vi "FRC_Scout.vi"() -> ()   [LabVIEW 2013]
doc: "The Grab (Express) VI acquires images continuously and displays the images in an image control using the Vision Acquisition Express VI. A grab is appropriate for high-speed applications in which you need to process only one image at a time."
uses:
  <vilib>/vision/Instrument.llb/QR Code Search Options.ctl
  <vilib>/vision/Instrument.llb/Demodulation Mode.ctl
  <vilib>/vision/Instrument.llb/Cell Sample Size.ctl
  <vilib>/vision/Instrument.llb/Cell Filter Mode.ctl
  <vilib>/vision/Instrument.llb/QR Code Description Options.ctl
  <vilib>/vision/Instrument.llb/Data Matrix Polarity.ctl
  <vilib>/vision/Instrument.llb/QR Code Model Type.ctl
  Instance           1 22Saved   Grab (Express) .vi
  <vilib>/LVH/i3 JSON/JSON Generation/Create Value Files/Create Value - Object.vi
  <vilib>/LVH/i3 JSON/JSON Generation/Add Object Parameter Files/Add Object Parameter - Object.vi
  <vilib>/LVH/i3 JSON/JSON Parsing/Get Object Parameter Files/Get Object Parameter - Object.vi
  <vilib>/vision/NI_Vision_Development_Module.lvlib
  <vilib>/LVH/i3 JSON/i3-json.lvlib
panel:
  out "Header":string
  out "Scores":T1
  out "Auto":T2
  out "Team":T3
  in  "QR Tab Control":T4(tab)
  in  "Auto Comments":string="How did autonomous work?"
  in  "T Stack":bool
  in  "B Mov":bool
  in  "T Mov":bool
  in  "Can PU Rec Bin":bool
  in  "Can PU Tote":bool
  in  "Can PU Noodles":bool
  in  "Drive Train":u16(ring) items=["Standard Wheels", "Omni Wheels", "Mecanum Wheels", "Swerve Drive"]
  in  "Comments":string="What else do we need to know?"
  in  "Max Tote":u8
  in  "Match":string="0"
  in  "Team #":u16
  in  "0":u8
  in  "1":u8
  in  "4":u8
  in  "2":u8
  in  "6A":u8
  in  "6B":u8
  in  "Inc0":bool
  in  "Inc1":bool
  in  "Inc2":bool
  in  "Inc4":bool
  in  "Inc6A":bool
  in  "Inc6B":bool
  in  "6C":u8
  in  "8":u8
  in  "10":u8
  in  "12A":u8
  in  "12B":u8
  in  "12C":u8
  in  "18A":u8
  in  "18B":u8
  in  "20":u8
  in  "24A":u8
  in  "24B":u8
  in  "30A":u8
  in  "30B":u8
  in  "36A":u8
  in  "36B":u8
  in  "40":u8
  in  "42":u8
  in  "Inc6C":bool
  in  "Inc8":bool
  in  "Inc10":bool
  in  "Inc12A":bool
  in  "Inc12B":bool
  in  "Inc12C":bool
  in  "Inc18B":bool
  in  "Inc18A":bool
  in  "Inc20":bool
  in  "Inc24A":bool
  in  "Inc24B":bool
  in  "Inc30A":bool
  in  "Inc30B":bool
  in  "Inc36A":bool
  in  "Inc36B":bool
  in  "Inc40":bool
  in  "Inc42":bool
  in  "Mov":bool
  out "Text Size":i32
  in  "Save  JSON":bool
  in  "Save Image":bool
  out "QR Code":picture
  out "output array":i8[][](array[numeric])
  in  "Export":enum16{"Off", "PNG", "EPS", "JPG"}(ring)=enum."JPG"
  in  "String":string
  in  "Stop Button":bool
  in  "Read New":bool
  out "Frame Rate":dbl
  out "Image":T5(plugin-control)
  out "Buffer Number":u32
  out "Message":string
  out "Read Time (ms)":dbl format="%.2f"
  out "QR Code \nfound":bool
  out "Valid \nRecord":bool
  in  "Save":bool
  out "Team":u16
  out "Match":string
  in  "Assemble and Save":bool
  out "File Number":i32
  in  "Stop":bool
  # "Match"
  # "No QR Code can be produced if \n                  is larger than 2740"
  # "Can pickup:"
  # "Robot Features"
  # "Scoring"
  # "Autonomous"
  # "Moved"
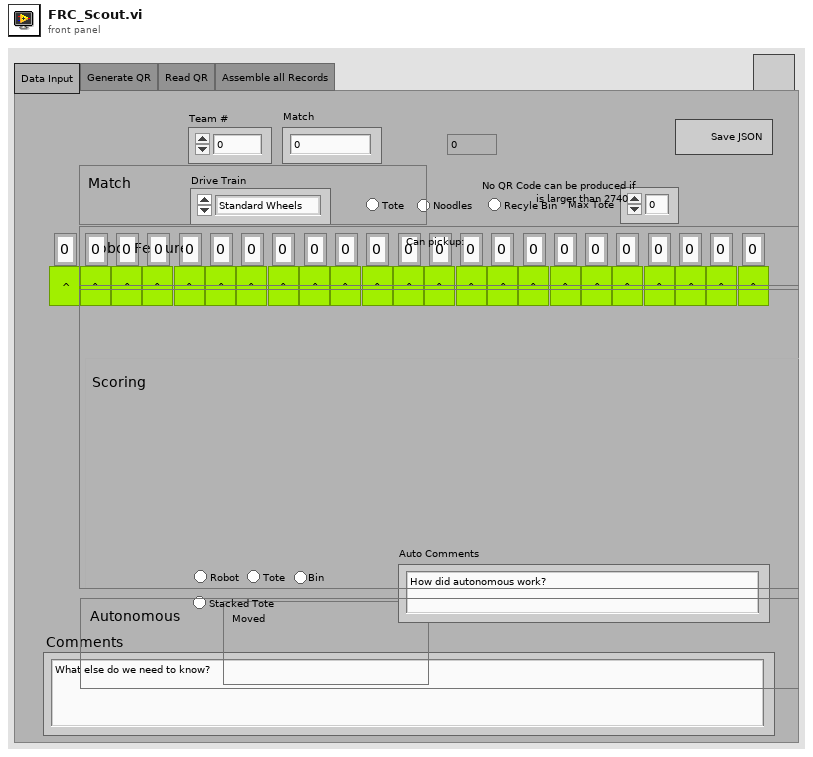
[diagram p1: front panel]
types:
  T1 = cluster{"0":u8, "1":u8, "2":u8, "4":u8, "6A":u8, "6B":u8, "6C":u8, "8":u8, "10":u8, "12A":u8, "12B":u8, "12C":u8, "18A":u8, "18B":u8, "20":u8, "24A":u8, "24B":u8, "30A":u8, "30B":u8, "36A":u8, "36B":u8, "40":u8, "42":u8}
  T2 = cluster{"Robot":bool, "Tote":bool, "Bin":bool, "Tote Stack":bool, "Auto Com":string}
  T3 = cluster{"Unique":string, "Team #":u16, "Match":string, "Max Tote":u8, "Drive":u16, "Noodles":bool, "Tote":bool, "Recylce Bin":bool, "Com":string}
  T4 = enum32{"Data Input", "Generate QR", "Read QR", "Assemble all Records"}
  T5 = typedef "IMAQ Image.ctl" = refnum<image>
  T6 = enum16{"Auto", "1", "2", "3", "4", "5", "6", "7", "8", "9", "10", "11", "12", "13", "14", "15", "16", "17", "18", "19", "20", "21", "22", "23", "24", "25", "26", "27", "28", "29", "30", "31", "32", "33", "34", "35", "36", "37", "38", "39", "40"}
  T7 = enum16{"Numeric", "Alphanumeric", "Binary", "Japanese"}
  T8 = typedef "Image Type" = u32
  T9 = typedef "QR Code Description Options.ctl" = cluster{"Matrix Size (cells)":i32, "Barcode Polarity":T10, "Mirror Mode":i32, "QR Model":T11}
  T10 = typedef "Data Matrix Polarity.ctl" = i32
  T11 = typedef "QR Code Model Type.ctl" = i32
  T12 = typedef "QR Code Search Options.ctl" = cluster{"Rotation Mode":enum32{"Unlimited", "0 Degrees", "90 Degrees", "180 Degrees", "270 Degrees"}, "Skip Location?":bool, "Edge Threshold":u32, "Demodulation Mode":T13, "Cell Sample Size":T14, "Cell Filter Mode":T15, "Skew Degrees Allowed":u32}
  T13 = typedef "Demodulation Mode.ctl" = i32
  T14 = typedef "Cell Sample Size.ctl" = i32
  T15 = typedef "Cell Filter Mode.ctl" = i32
  T16 = typedef "QR Code Report.ctl" = cluster{"Found?":bool, "Data":string, "Bounding Box":cluster{"x":sgl, "y":sgl}[], "Errors Corrected":u32, "Dimensions (Rows/Cols)":u32, "Version":u32, "QR Model":T11, "Stream Mode":T17, "Barcode Polarity":T10, "Mirrored?":bool, "Append Stream Position":u32, "Size of Append Stream":u32, "First EAN-128 ID":i32, "First Alternate Language ID":i32, "Append Stream ID":u32, "Minimum Edge Strength":u32, "Demodulation Mode":T13, "Cell Sample Size":T14, "Cell Filter Mode":T15}
  T17 = typedef "QR Code Stream Mode Type.ctl" = i32
  T18 = cluster{"Unique":string, "Team #":u16, "Match":string, "Max Tote":u8, "Drive Train":u16, "Can PU Noodles":bool, "Can PU Tote":bool, "Can PU Rec Bin":bool, "Comments":string}
  T19 = cluster{"Mov":bool, "T Mov":bool, "B Mov":bool, "T Stack":bool, "Auto Comments":string}
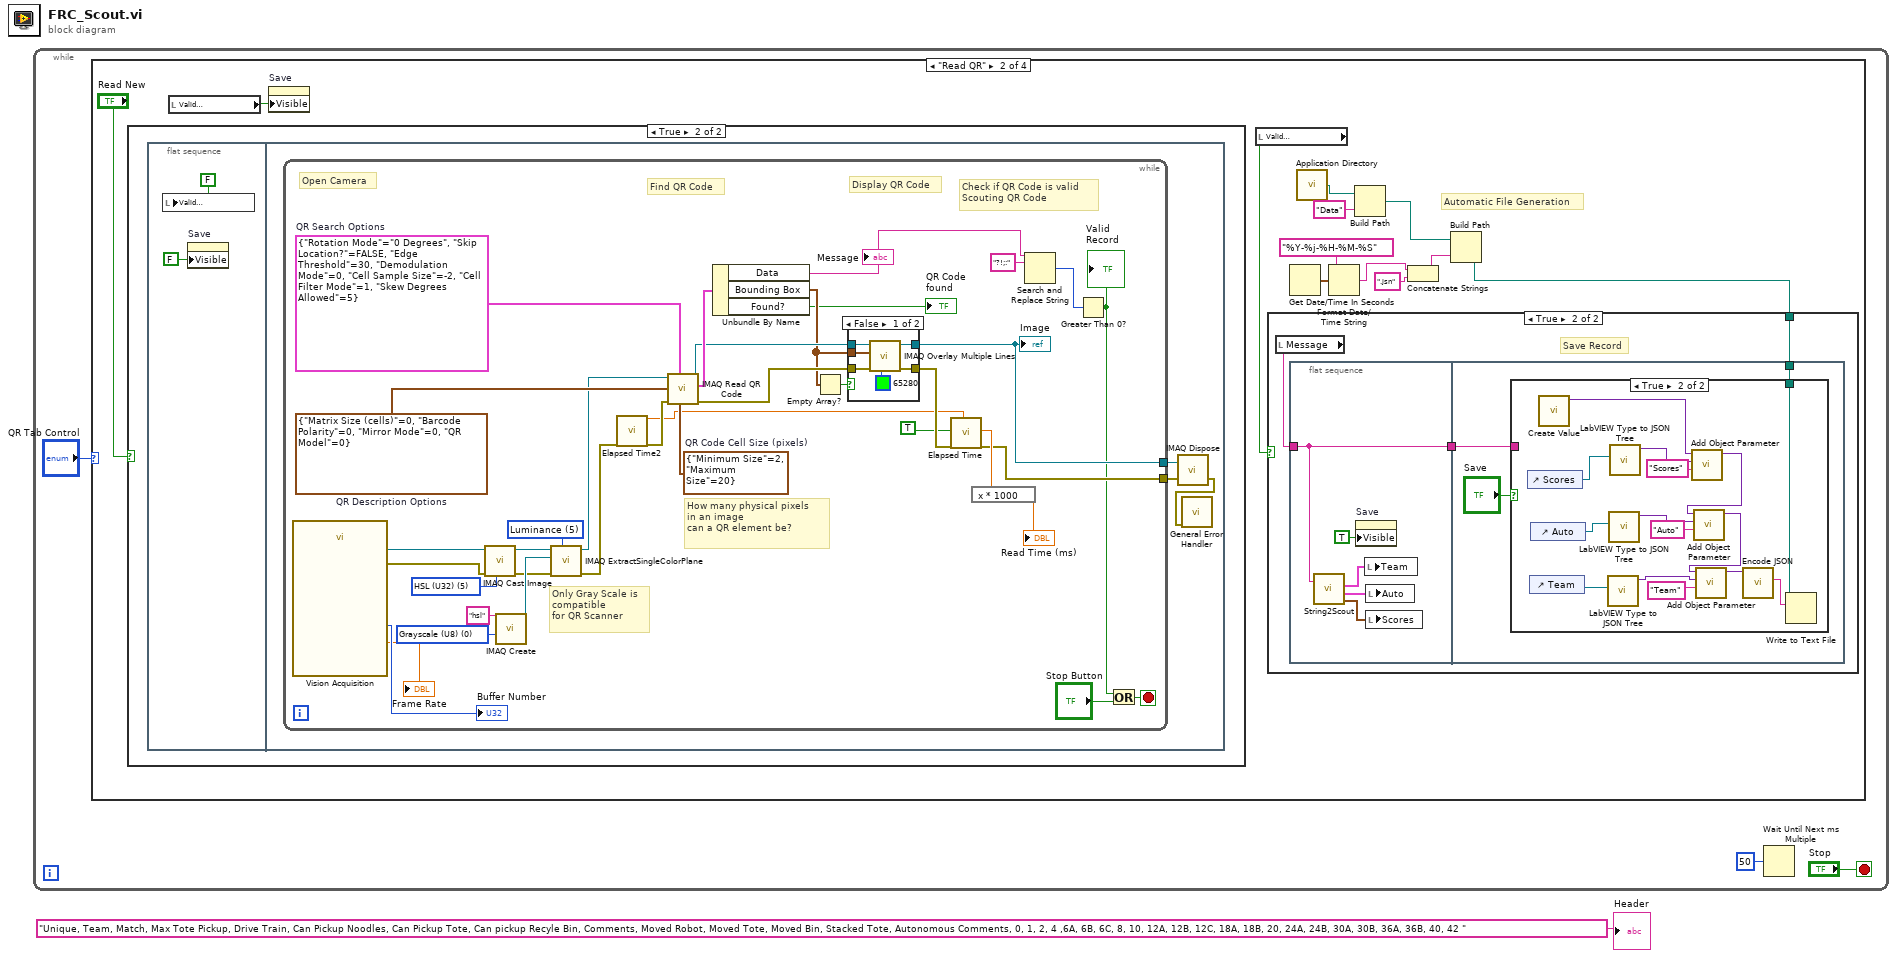
[diagram p0: block diagram]
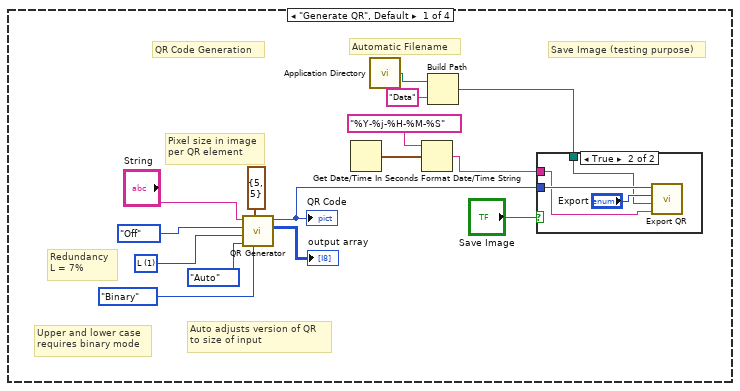
[diagram p2: hidden frame]
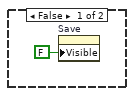
[diagram p4: hidden frame]
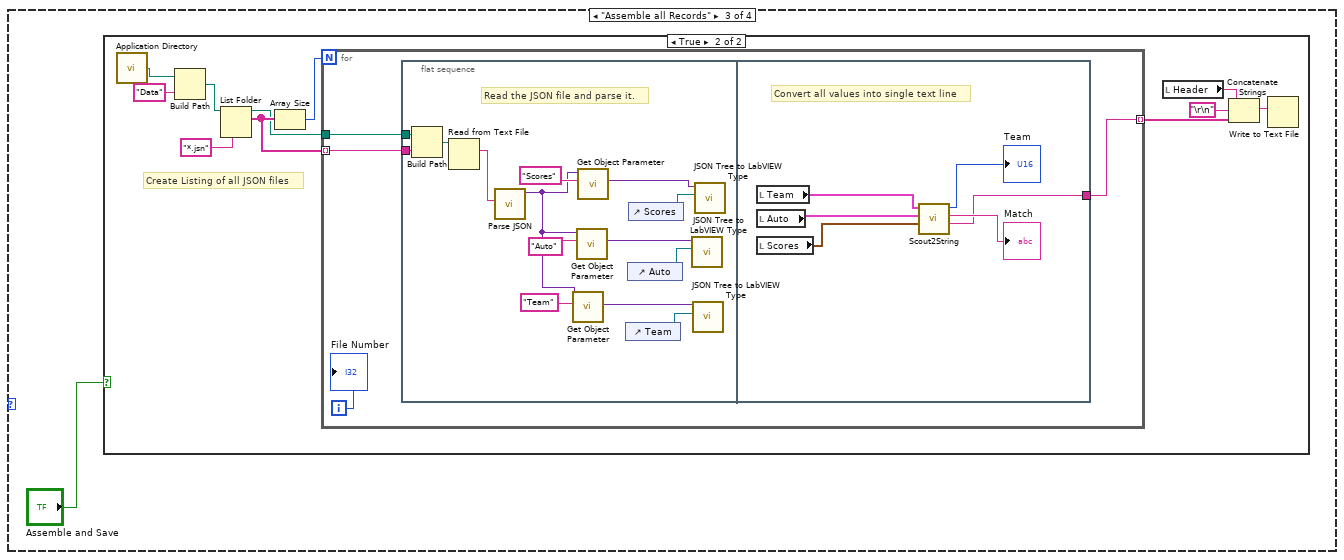
[diagram p8: hidden frame]
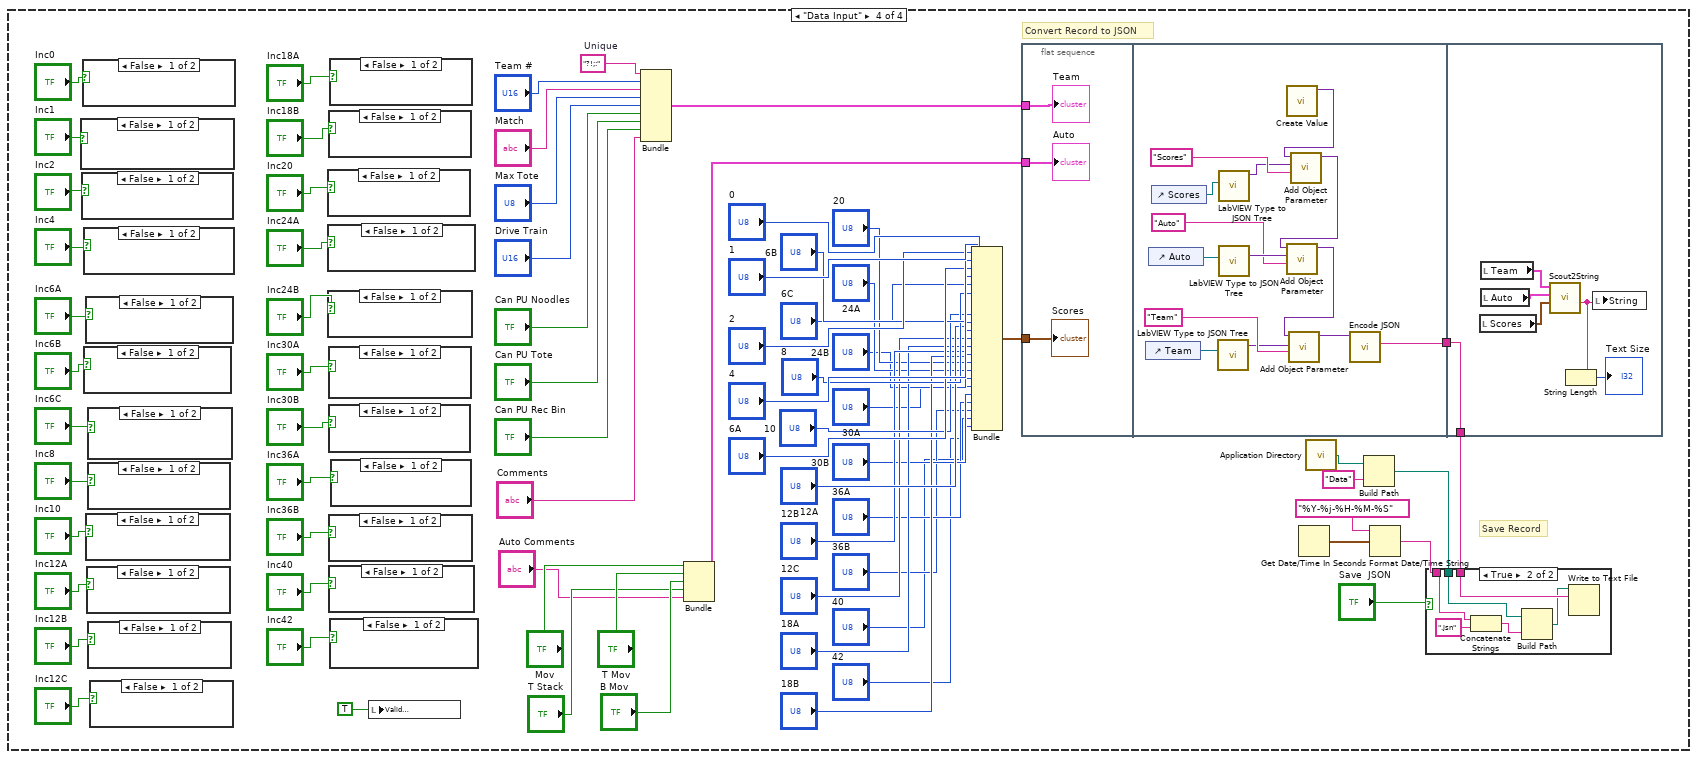
[diagram p10: hidden frame]
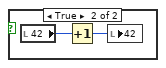
[diagram p12: hidden frame]
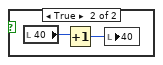
[diagram p13: hidden frame]
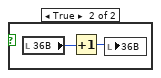
[diagram p14: hidden frame]
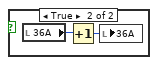
[diagram p15: hidden frame]
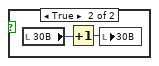
[diagram p16: hidden frame]
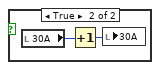
[diagram p17: hidden frame]
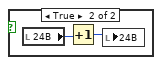
[diagram p18: hidden frame]
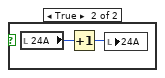
[diagram p19: hidden frame]
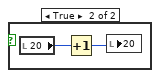
[diagram p20: hidden frame]
diagram:
  n1 = while {
    stop <- "Stop" stop-if-true
    n2 = case shown="\"Read QR\"" "QR Tab Control" {
      frame "Generate QR", Default {
        w17 = u16 1 items=["L"=1, "M"=0, "Q"=3, "H"=2] ("Error Correction")
        # "Pixel size in image\nper QR element"
        # "Auto adjusts version of QR\nto size of input"
        # "Upper and lower case\nrequires binary mode"
        # "Redundancy\nL = 7%"
        # "Save Image (testing purpose)"
        # "QR Code Generation"
        # "Automatic Filename"
        n3 = call "QR Generator.vi"("Data Mode"=T7."Binary", "Size"=cluster{"Width":i32, "Height":i32} {"Width"=5, "Height"=5}, "Version"=T6."Auto", "Error Correction"=w17, "Export"=enum16{"Off", "PNG", "EPS", "JPG"}."Off", "Message"="String") -> ("output array"=→"output array":i8[][], "QR Code"=w14:picture)  [unwired: 4 in]
        "QR Code" <- w14
        n4 = Get Date/Time In Seconds() -> (seconds since 1Jan1904=w8:timestamp)
        n5 = call <vilib>:"Application Directory.vi"() -> ("Application Directory"=w12:path)
        n6 = Format Date/Time String(time format string (%c)="%Y-%j-%H-%M-%S", seconds (now)=w8) -> (date/time string=w7:string)  [unwired: 1 in]
        n7 = Build Path(base path=w12, name or relative path="Data") -> (appended path=w10:path)
        n8 = case shown="True" "Save Image" {
          tunnel: w14 -> [_ w23]
          tunnel: w10 -> [_ w21]
          tunnel: w7 -> [_ w20]
          frame False {
          }
          frame True {
            n9 = call "Export QR.vi"("File Name"=w20, "path to graphics file"=w21, "Export"="Export", "Picture"=w23) -> ()  [unwired: 8 in]
          }
        }
      }
      frame "Read QR" {
        # "Automatic File Generation"
        n10 = case shown="True" "Read New" {
          frame False {
          }
          frame True {
            n11 = flat-sequence {
              frame #0 {
                n12 = local write "Valid \nRecord"(FALSE ("Valid QR \nCode found")) -> ()
                n13 = property on="Save" class="Bool"("Visible"=FALSE) -> ()  [unwired: 2 in, 2 out]
              }
              frame #1 {
                n14 = while {
                  tunnel: [w76] -> w67
                  tunnel: [w75] -> w66
                  stop <- w71 stop-if-true
                  w89 = T8 0 items=["Grayscale (U8)", "Grayscale (I16)", "Grayscale (SGL)", "Complex (CSG)", "RGB (U32)", "HSL (U32)", "RGB (U64)", "Grayscale (U16)"] ("Image Type")
                  w90 = 5 items=["Red", "Green", "Blue", "Hue", "Saturation", "Luminance", "Value", "Intensity"] ("Color Plane")
                  w92 = T8 5 items=["Grayscale (U8)", "Grayscale (I16)", "Grayscale (SGL)", "Complex (CSG)", "RGB (U32)", "HSL (U32)", "RGB (U64)", "Grayscale (U16)"] ("Image Type")
                  w96 = cluster{"Minimum Size":u32, "Maximum Size":u32} {"Minimum Size"=2, "Maximum Size"=20}  # QR Code Cell Size (pixels)
                  w100 = T9 {"Matrix Size (cells)"=0, "Barcode Polarity"=0, "Mirror Mode"=0, "QR Model"=0}  # QR Description Options
                  w101 = T12 {"Rotation Mode"=enum."0 Degrees", "Skip Location?"=FALSE, "Edge Threshold"=30, "Demodulation Mode"=0, "Cell Sample Size"=-2, "Cell Filter Mode"=1, "Skew Degrees Allowed"=5}  # QR Search Options
                  # "How many physical pixels \nin an image\ncan a QR element be?"
                  # "Only Gray Scale is \ncompatible \nfor QR Scanner"
                  # "Check if QR Code is valid \nScouting QR Code"
                  # "Display QR Code"
                  # "Find QR Code"
                  # "Open Camera"
                  n15 = call "Vision Acquisition"() -> ("Image Out"=w87:T5, "Image Number"=→"Buffer Number":u32, "Frame Rate"=→"Frame Rate":dbl, "error out"=w86:errorcluster)  [unwired: 2 in, 22 out]
                  n16 = call "IMAQ Cast Image"("Image Type"=w92, "error in (no error)"=w86, "Image Src"=w87) -> ("error out"=w84:errorcluster, "Image Dst Out"=w91:T5)  [unwired: 7 in]
                  n17 = call "IMAQ Create"("Image Name"="hsl", "Image Type"=w89) -> ("New Image"=w88:T5)  [unwired: 3 in, 1 out]
                  n18 = call "IMAQ ExtractSingleColorPlane"("Color Plane"=w90, "error in (no error)"=w84, "Image Dst"=w88, "Image Src"=w91) -> ("error out"=w83:errorcluster, "Image Dst Out"=w85:T5)  [unwired: 6 in]
                  n19 = call "Elapsed Time2"("error in (no error)"=w83) -> ("Present (s)"=w77:dbl, "error out"=w95:errorcluster)  [unwired: 11 in, 6 out]
                  n20 = call "IMAQ Read QR Code"("QR Code Cell Size (pixels)"=w96, "QR Search Options"=w101, "error in (no error)"=w95, "QR Description Options"=w100, "Image"=w85) -> ("error out"=w97:errorcluster, "QR Code Report"=w99:T16, "Image (duplicate)"=w98:T5)  [unwired: 3 in, 1 out]
                  n21 = Unbundle By Name(w99) -> ("Data"=w68:string, "Bounding Box"=w81:cluster{"x":sgl, "y":sgl}[], "Found?"=→"QR Code \nfound":bool)
                  "Message" <- w68
                  n22 = Empty Array?(array=w81) -> (empty?=w80:bool)
                  n23 = case shown="False" w80 {
                    tunnel: w98 -> [w109 w111]
                    tunnel: w97 -> [w108 w110]
                    tunnel: [w106 w110] -> w94
                    tunnel: w81 -> [w105 _]
                    tunnel: [w104 w111] -> w76
                    frame False {
                      n24 = call "IMAQ Overlay Multiple Lines"("Color"=u32 65280, "error in (no error)"=w108, "Line End Points"=w105, "Image"=w109) -> ("error out"=w106:errorcluster, "Image Out"=w104:T5)  [unwired: 6 in]
                    }
                    frame True {
                    }
                  }
                  "Image" <- w76
                  n25 = call "Elapsed Time"("Reset"=TRUE, "error in (no error)"=w94, "Set Start Time (s)"=w77) -> ("Elapsed Time (s)"=w78:dbl, "error out"=w75:errorcluster)  [unwired: 9 in, 6 out]
                  n26 = expression code="x * 1000"(w78) -> (→"Read Time (ms)":dbl)
                  n27 = Search and Replace String(input string=w68, search string="?!;:") -> (number of replacements=w72:i32)  [unwired: 6 in, 3 out]
                  n28 = Greater Than 0?(x=w72) -> (x > 0?=w70:bool)
                  "Valid \nRecord" <- w70
                  n29 = Or(x=w70, y="Stop Button") -> (x .or. y?=w71:bool)
                }
                n30 = call "IMAQ Dispose"("Image"=w67, "error in (no error)"=w66) -> ("error out"=w65:errorcluster)  [unwired: 4 in]
                n31 = call <vilib>:"General Error Handler.vi"("error in (no error)"=w65) -> ()  [unwired: 1 in, 14 out]
              }
            }
          }
        }
        n32 = local read "Valid \nRecord"() -> (w24:bool)
        n33 = property on="Save" class="Bool"("Visible"=w24) -> ()  [unwired: 2 in, 2 out]
        n34 = local read "Valid \nRecord"() -> (w25:bool)
        n35 = Get Date/Time In Seconds() -> (seconds since 1Jan1904=w32:timestamp)
        n36 = call <vilib>:"Application Directory.vi"() -> ("Application Directory"=w35:path)
        n37 = Format Date/Time String(time format string (%c)="%Y-%j-%H-%M-%S", seconds (now)=w32) -> (date/time string=w28:string)  [unwired: 1 in]
        n38 = Build Path(base path=w35, name or relative path="Data") -> (appended path=w31:path)
        n39 = Concatenate Strings(w28, ".jsn" ("string")) -> (w27:string)
        n40 = Build Path(base path=w31, name or relative path=w27) -> (appended path=w30:path)
        n41 = case shown="True" w25 {
          tunnel: w30 -> [_ w39]
          frame False {
            n42 = property on="Save" class="Bool"("Visible"=FALSE) -> ()  [unwired: 2 in, 2 out]
          }
          frame True {
            # "Save Record"
            n43 = local read "Message"() -> (w38:string)
            n44 = flat-sequence {
              tunnel: w38 -> [w40]
              tunnel: [w40] -> w37
              tunnel: w39 -> [w46]
              tunnel: w37 -> [w45]
              frame #0 {
                n45 = call "String2Scout.vi"("String"=w40) -> ("Team Out"=w42:T3, "Auto Out"=w43:T2, "Scores Out"=w44:T1)  [unwired: 1 in, 3 out]
                n46 = property on="Save" class="Bool"("Visible"=TRUE) -> ()  [unwired: 2 in, 2 out]
                n47 = local write "Team"(w42) -> ()
                n48 = local write "Auto"(w43) -> ()
                n49 = local write "Scores"(w44) -> ()
              }
              frame #1 {
                n50 = case shown="True" "Save" {
                  tunnel: w45 -> [_ _]
                  tunnel: w46 -> [_ w62]
                  frame False {
                  }
                  frame True {
                    n51 = control-ref of="Scores"() -> (w48:refnum<vi>)
                    n52 = control-ref of="Team"() -> (w50:refnum<vi>)
                    n53 = control-ref of="Auto"() -> (w49:refnum<vi>)
                    n54 = call-poly <vilib>:"Create Value.vi"() -> ("JSON Tree"=w57:variant)  [unwired: 10 in, 1 out]
                    n55 = call <vilib>:"LabVIEW Type to JSON Tree.vi"("Ctl Refnum"=w50) -> ("JSON Tree Out"=w53:variant)  [unwired: 9 in, 1 out]
                    n56 = call <vilib>:"LabVIEW Type to JSON Tree.vi"("Ctl Refnum"=w49) -> ("JSON Tree Out"=w52:variant)  [unwired: 9 in, 1 out]
                    n57 = call <vilib>:"LabVIEW Type to JSON Tree.vi"("Ctl Refnum"=w48) -> ("JSON Tree Out"=w51:variant)  [unwired: 9 in, 1 out]
                    n58 = call-poly <vilib>:"Add Object Parameter.vi"("Name"="Scores", "JSON Object"=w51, "JSON Tree in (JSON Object)"=w57) -> ("JSON Tree out (JSON Object)"=w56:variant)  [unwired: 7 in, 1 out]
                    n59 = call-poly <vilib>:"Add Object Parameter.vi"("Name"="Auto", "JSON Object"=w52, "JSON Tree in (JSON Object)"=w56) -> ("JSON Tree out (JSON Object)"=w55:variant)  [unwired: 7 in, 1 out]
                    n60 = call-poly <vilib>:"Add Object Parameter.vi"("Name"="Team", "JSON Object"=w53, "JSON Tree in (JSON Object)"=w55) -> ("JSON Tree out (JSON Object)"=w54:variant)  [unwired: 7 in, 1 out]
                    n61 = call <vilib>:"Encode JSON.vi"("JSON Tree"=w54) -> ("String"=w61:string)  [unwired: 5 in, 1 out]
                    n62 = Write to Text File(file (use dialog)=w62, text=w61) -> ()  [unwired: 2 in, 3 out]
                  }
                }
              }
            }
          }
        }
      }
      frame "Assemble all Records" {
        n63 = case shown="True" "Assemble and Save" {
          frame False {
          }
          frame True {
            # "Create Listing of all JSON files"
            n64 = call <vilib>:"Application Directory.vi"() -> ("Application Directory"=w123:path)
            n65 = Build Path(base path=w123, name or relative path="Data") -> (appended path=w121:path)
            n66 = List Folder(path=w121, pattern="*.jsn") -> (path out=w117:path, filenames=w118:string[])  [unwired: 2 in, 2 out]
            n67 = Array Size(array=w118) -> (size(s)=w119:i32)
            n68 = for {
              N: w119 -> [_]
              tunnel: w118 -> [w126] mode=indexing
              tunnel: w117 -> [w127]
              tunnel: [w124] -> w113 mode=indexing
              i -> [w125]
              n69 = flat-sequence {
                tunnel: w127 -> [w141]
                tunnel: w126 -> [w140]
                tunnel: [w142] -> w124
                frame #0 {
                  # "Read the JSON file and parse it."
                  n70 = Build Path(base path=w141, name or relative path=w140) -> (appended path=w139:path)
                  n71 = Read from Text File(file (use dialog)=w139) -> (text=w136:string)  [unwired: 3 in, 3 out]
                  n72 = call <vilib>:"Parse JSON.vi"("JSON String"=w136) -> ("JSON Tree"=w135:variant)  [unwired: 7 in, 3 out]
                  n73 = call-poly <vilib>:"Get Object Parameter.vi"("Parameter Name"="Team", "JSON Tree In (JSON Object)"=w135) -> ("JSON Object"=w130:variant)  [unwired: 6 in, 3 out]
                  n74 = call-poly <vilib>:"Get Object Parameter.vi"("Parameter Name"="Auto", "JSON Tree In (JSON Object)"=w135) -> ("JSON Object"=w131:variant)  [unwired: 6 in, 3 out]
                  n75 = call-poly <vilib>:"Get Object Parameter.vi"("Parameter Name"="Scores", "JSON Tree In (JSON Object)"=w135) -> ("JSON Object"=w133:variant)  [unwired: 6 in, 3 out]
                  n76 = control-ref of="Team"() -> (w129:refnum<vi>)
                  n77 = control-ref of="Auto"() -> (w128:refnum<vi>)
                  n78 = control-ref of="Scores"() -> (w132:refnum<vi>)
                  n79 = call <vilib>:"JSON Tree to LabVIEW Type.vi"("Ctl Refnum"=w128, "JSON Tree In"=w131) -> ()  [unwired: 8 in, 2 out]
                  n80 = call <vilib>:"JSON Tree to LabVIEW Type.vi"("Ctl Refnum"=w129, "JSON Tree In"=w130) -> ()  [unwired: 8 in, 2 out]
                  n81 = call <vilib>:"JSON Tree to LabVIEW Type.vi"("Ctl Refnum"=w132, "JSON Tree In"=w133) -> ()  [unwired: 8 in, 2 out]
                }
                frame #1 {
                  # "Convert all values into single text line"
                  n82 = local read "Team"() -> (w145:T3)
                  n83 = local read "Auto"() -> (w144:T2)
                  n84 = local read "Scores"() -> (w143:T1)
                  n85 = call "Scout2String.vi"("Scores"=w143, "Auto"=w144, "Team"=w145) -> ("String"=w142:string, "Match"=→"Match":string, "Team"=→"Team":u16)  [unwired: 6 in]
                }
              }
              "File Number" <- w125
            }
            n86 = local read "Header"() -> (w114:string)
            n87 = Concatenate Strings(w114, "\r\n", w113) -> (w116:string)
            n88 = Write to Text File(text=w116) -> ()  [unwired: 3 in, 3 out]
          }
        }
      }
      frame "Data Input" {
        w152 = "?!;:"  # Unique
        # "Convert Record to JSON"
        # "Save Record"
        n89 = case shown="False" "Inc1" {
          frame False {
          }
          frame True {
            n90 = local read "1"() -> (w292:u8)
            n91 = Increment(x=w292) -> (x+1=w293:u8)
            n92 = local write "1"(w293) -> ()
          }
        }
        n93 = case shown="False" "Inc2" {
          frame False {
          }
          frame True {
            n94 = local read "2"() -> (w291:u8)
            n95 = Increment(x=w291) -> (x+1=w290:u8)
            n96 = local write "2"(w290) -> ()
          }
        }
        n97 = case shown="False" "Inc0" {
          frame False {
          }
          frame True {
            n98 = local read "0"() -> (w295:u8)
            n99 = Increment(x=w295) -> (x+1=w294:u8)
            n100 = local write "0"(w294) -> ()
          }
        }
        n101 = case shown="False" "Inc4" {
          frame False {
          }
          frame True {
            n102 = local read "4"() -> (w289:u8)
            n103 = Increment(x=w289) -> (x+1=w288:u8)
            n104 = local write "4"(w288) -> ()
          }
        }
        n105 = case shown="False" "Inc6B" {
          frame False {
          }
          frame True {
            n106 = local read "6B"() -> (w285:u8)
            n107 = Increment(x=w285) -> (x+1=w284:u8)
            n108 = local write "6B"(w284) -> ()
          }
        }
        n109 = case shown="False" "Inc6A" {
          frame False {
          }
          frame True {
            n110 = local read "6A"() -> (w287:u8)
            n111 = Increment(x=w287) -> (x+1=w286:u8)
            n112 = local write "6A"(w286) -> ()
          }
        }
        n113 = case shown="False" "Inc10" {
          frame False {
          }
          frame True {
            n114 = local read "10"() -> (w279:u8)
            n115 = Increment(x=w279) -> (x+1=w278:u8)
            n116 = local write "10"(w278) -> ()
          }
        }
        n117 = case shown="False" "Inc12A" {
          frame False {
          }
          frame True {
            n118 = local read "12A"() -> (w276:u8)
            n119 = Increment(x=w276) -> (x+1=w277:u8)
            n120 = local write "12A"(w277) -> ()
          }
        }
        n121 = case shown="False" "Inc6C" {
          frame False {
          }
          frame True {
            n122 = local read "6C"() -> (w283:u8)
            n123 = Increment(x=w283) -> (x+1=w282:u8)
            n124 = local write "6C"(w282) -> ()
          }
        }
        n125 = case shown="False" "Inc8" {
          frame False {
          }
          frame True {
            n126 = local read "8"() -> (w280:u8)
            n127 = Increment(x=w280) -> (x+1=w281:u8)
            n128 = local write "8"(w281) -> ()
          }
        }
        n129 = case shown="False" "Inc12B" {
          frame False {
          }
          frame True {
            n130 = local read "12B"() -> (w275:u8)
            n131 = Increment(x=w275) -> (x+1=w274:u8)
            n132 = local write "12B"(w274) -> ()
          }
        }
        n133 = case shown="False" "Inc12C" {
          frame False {
          }
          frame True {
            n134 = local read "12C"() -> (w272:u8)
            n135 = Increment(x=w272) -> (x+1=w273:u8)
            n136 = local write "12C"(w273) -> ()
          }
        }
        n137 = case shown="False" "Inc20" {
          frame False {
          }
          frame True {
            n138 = local read "20"() -> (w266:u8)
            n139 = Increment(x=w266) -> (x+1=w267:u8)
            n140 = local write "20"(w267) -> ()
          }
        }
        n141 = case shown="False" "Inc24A" {
          frame False {
          }
          frame True {
            n142 = local read "24A"() -> (w264:u8)
            n143 = Increment(x=w264) -> (x+1=w265:u8)
            n144 = local write "24A"(w265) -> ()
          }
        }
        n145 = case shown="False" "Inc24B" {
          frame False {
          }
          frame True {
            n146 = local read "24B"() -> (w262:u8)
            n147 = Increment(x=w262) -> (x+1=w263:u8)
            n148 = local write "24B"(w263) -> ()
          }
        }
        n149 = case shown="False" "Inc18B" {
          frame False {
          }
          frame True {
            n150 = local read "18B"() -> (w268:u8)
            n151 = Increment(x=w268) -> (x+1=w269:u8)
            n152 = local write "18B"(w269) -> ()
          }
        }
        n153 = case shown="False" "Inc30A" {
          frame False {
          }
          frame True {
            n154 = local read "30A"() -> (w260:u8)
            n155 = Increment(x=w260) -> (x+1=w261:u8)
            n156 = local write "30A"(w261) -> ()
          }
        }
        n157 = case shown="False" "Inc30B" {
          frame False {
          }
          frame True {
            n158 = local read "30B"() -> (w258:u8)
            n159 = Increment(x=w258) -> (x+1=w259:u8)
            n160 = local write "30B"(w259) -> ()
          }
        }
        n161 = case shown="False" "Inc36B" {
          frame False {
          }
          frame True {
            n162 = local read "36B"() -> (w254:u8)
            n163 = Increment(x=w254) -> (x+1=w255:u8)
            n164 = local write "36B"(w255) -> ()
          }
        }
        n165 = case shown="False" "Inc40" {
          frame False {
          }
          frame True {
            n166 = local read "40"() -> (w252:u8)
            n167 = Increment(x=w252) -> (x+1=w253:u8)
            n168 = local write "40"(w253) -> ()
          }
        }
        n169 = case shown="False" "Inc18A" {
          frame False {
          }
          frame True {
            n170 = local read "18A"() -> (w270:u8)
            n171 = Increment(x=w270) -> (x+1=w271:u8)
            n172 = local write "18A"(w271) -> ()
          }
        }
        n173 = case shown="False" "Inc42" {
          frame False {
          }
          frame True {
            n174 = local read "42"() -> (w250:u8)
            n175 = Increment(x=w250) -> (x+1=w251:u8)
            n176 = local write "42"(w251) -> ()
          }
        }
        n177 = case shown="False" "Inc36A" {
          frame False {
          }
          frame True {
            n178 = local read "36A"() -> (w256:u8)
            n179 = Increment(x=w256) -> (x+1=w257:u8)
            n180 = local write "36A"(w257) -> ()
          }
        }
        n181 = local write "Valid \nRecord"(TRUE ("Valid QRC found")) -> ()
        n182 = Bundle("Unique"=w152, "Team #"="Team #", "Match"="Match", "Max Tote"="Max Tote", "Drive Train"="Drive Train", "Can PU Noodles"="Can PU Noodles", "Can PU Tote"="Can PU Tote", "Can PU Rec Bin"="Can PU Rec Bin", "Comments"="Comments") -> (w184:T18)  [unwired: 1 in]
        n183 = Bundle("Mov"="Mov", "T Mov"="T Mov", "B Mov"="B Mov", "T Stack"="T Stack", "Auto Comments"="Auto Comments") -> (w183:T19)  [unwired: 1 in]
        n184 = Bundle("0"="0", "1"="1", "2"="2", "4"="4", "6A"="6A", "6B"="6B", "6C"="6C", "8"="8", "10"="10", "12A"="12A", "12B"="12B", "12C"="12C", "18A"="18A", "18B"="18B", "20"="20", "24A"="24A", "24B"="24B", "30A"="30A", "30B"="30B", "36A"="36A", "36B"="36B", "40"="40", "42"="42") -> (w150:T1)  [unwired: 1 in]
        n185 = flat-sequence {
          tunnel: w184 -> [w223]
          tunnel: w183 -> [w221]
          tunnel: w150 -> [w222]
          tunnel: [w233] -> w149
          tunnel: [w243] -> w148
          tunnel: w149 -> [w243]
          frame #0 {
            "Team" <- w223
            "Auto" <- w221
            "Scores" <- w222
          }
          frame #1 {
            n186 = control-ref of="Team"() -> (w237:refnum<vi>)
            n187 = control-ref of="Auto"() -> (w235:refnum<vi>)
            n188 = control-ref of="Scores"() -> (w236:refnum<vi>)
            n189 = call <vilib>:"LabVIEW Type to JSON Tree.vi"("Ctl Refnum"=w237) -> ("JSON Tree Out"=w228:variant)  [unwired: 9 in, 1 out]
            n190 = call <vilib>:"LabVIEW Type to JSON Tree.vi"("Ctl Refnum"=w236) -> ("JSON Tree Out"=w229:variant)  [unwired: 9 in, 1 out]
            n191 = call <vilib>:"LabVIEW Type to JSON Tree.vi"("Ctl Refnum"=w235) -> ("JSON Tree Out"=w234:variant)  [unwired: 9 in, 1 out]
            n192 = call-poly <vilib>:"Create Value.vi"() -> ("JSON Tree"=w227:variant)  [unwired: 10 in, 1 out]
            n193 = call-poly <vilib>:"Add Object Parameter.vi"("Name"="Scores", "JSON Object"=w229, "JSON Tree in (JSON Object)"=w227) -> ("JSON Tree out (JSON Object)"=w226:variant)  [unwired: 7 in, 1 out]
            n194 = call-poly <vilib>:"Add Object Parameter.vi"("Name"="Auto", "JSON Object"=w234, "JSON Tree in (JSON Object)"=w226) -> ("JSON Tree out (JSON Object)"=w225:variant)  [unwired: 7 in, 1 out]
            n195 = call-poly <vilib>:"Add Object Parameter.vi"("Name"="Team", "JSON Object"=w228, "JSON Tree in (JSON Object)"=w225) -> ("JSON Tree out (JSON Object)"=w224:variant)  [unwired: 7 in, 1 out]
            n196 = call <vilib>:"Encode JSON.vi"("JSON Tree"=w224) -> ("String"=w233:string)  [unwired: 5 in, 1 out]
          }
          frame #2 {
            n197 = local read "Scores"() -> (w240:T1)
            n198 = local read "Team"() -> (w242:T3)
            n199 = local read "Auto"() -> (w241:T2)
            n200 = call "Scout2String.vi"("Scores"=w240, "Auto"=w241, "Team"=w242) -> ("String"=w238:string)  [unwired: 6 in, 2 out]
            n201 = String Length(string=w238) -> (length=→"Text Size":i32)
            n202 = local write "String"(w238) -> ()
          }
        }
        n203 = Get Date/Time In Seconds() -> (seconds since 1Jan1904=w153:timestamp)
        n204 = call <vilib>:"Application Directory.vi"() -> ("Application Directory"=w159:path)
        n205 = Build Path(base path=w159, name or relative path="Data") -> (appended path=w156:path)
        n206 = Format Date/Time String(time format string (%c)="%Y-%j-%H-%M-%S", seconds (now)=w153) -> (date/time string=w154:string)  [unwired: 1 in]
        n207 = case shown="True" "Save  JSON" {
          tunnel: w148 -> [_ w245]
          tunnel: w156 -> [_ w249]
          tunnel: w154 -> [_ w246]
          frame False {
          }
          frame True {
            n208 = Concatenate Strings(w246, ".jsn" ("string")) -> (w248:string)
            n209 = Build Path(base path=w249, name or relative path=w248) -> (appended path=w244:path)
            n210 = Write to Text File(file (use dialog)=w244, text=w245) -> ()  [unwired: 2 in, 3 out]
          }
        }
      }
    }
    n211 = Wait Until Next ms Multiple(millisecond multiple=u32 50) -> ()  [unwired: 1 out]
  }
  "Header" <- "Unique, Team, Match, Max Tote Pickup, Drive Train, Can Pickup Noodles, Can Pickup Tote, Can pickup Recyle Bin, Comments, Moved Robot, Moved Tote, Moved Bin, Stacked Tote, Autonomous Comments, 0, 1, 2, 4 ,6A, 6B, 6C, 8, 10, 12A, 12B, 12C, 18A, 18B, 20, 24A, 24B, 30A, 30B, 36A, 36B, 40, 42 " ("string")
